vi "Global_usbComm.vi"() -> ()   [LabVIEW 2018]
panel:
  in  "Inspection Point":string
  in  "Specsheet Scan":string
  in  "PO Line Number":string
  in  "PO Number":string
  in  "Inspector":string="id:0"
  in  "Station":string
  in  "Serial Port":refnum<visa-resource-name>
  in  "Vendor Number":string
  in  "Vendor Name":string
  out "PIC_ARRAY":picture[](array[picture])=[bytes[1209480], bytes[921630], bytes[921630], bytes[346830], bytes[720330]]
  out "usbType":string
  out "Version":string[][](array[string])=[["Date", "Version", "Status", "Mod By"], ["20190701", "0", "Sic parvis magna", "id:0"], ["20191212", "1", "Successful test on 5 various consoles", "id:0"], ["20200125", "2", "Test for release", "id:0"], ["20200211", "3", "Fixed several bugs and rease for testing", "id:0"], ["20200213", "4", "Set foundation to handle Freemotion", "id:0"], ["20200214", "5", "Fixed small bugs", "id:0"], ["20200228", "6", "Changed reports so that all data will be visible with  SQL server", "id:0"], ["", "", "", ""]]
  in  "RS485_GearValues":dbl[][](array[numeric])=[[194.0, 245.0, 310.0, 375.0, 439.0, 504.0, 569.0, 634.0, 698.0, 763.0, 828.0, 892.0, 957.0, 1022.0, 1087.0, 1151.0, 1216.0, 1281.0, 1345.0, 1410.0, 1475.0, 1539.0, 0.0, 0.0, 0.0, 0.0], [194.0, 245.0, 310.0, 362.0, 427.0, 478.0, 543.0, 595.0, 659.0, 711.0, 776.0, 841.0, 892.0, 957.0, 1009.0, 1074.0, 1125.0, 1190.0, 1242.0, 1307.0, 1371.0, 1423.0, 1488.0, 1539.0, 0.0, 0.0], [194.0, 0.0, 0.0, 0.0, 0.0, 0.0, 0.0, 0.0, 0.0, 0.0, 0.0, 0.0, 0.0, 0.0, 0.0, 0.0, 0.0, 0.0, 0.0, 0.0, 0.0, 0.0, 0.0, 0.0, 0.0, 0.0]]
  out "resistanceType":string
  out "gradeType":string
  out "speedType":string
  out "tabletType":string
  in  "KeyCodes":string[][](array[string])=[["1", "2", "3", "4", "5", "6", "7", "8", "9", "10", "11", "12", "13", "14", "15", "", "", "", "", "", "", "", "", "", "", "", "", "", "", "", "", "", "", "", "", "", "", "", "", "", "", "", "", "", "", "", "", "", "", "", "", "", "", "", "", "", "", "", "", "", ""], ["1", "2", "3", "4", "5", "6", "7", "8", "9", "10", "11", "12", "13", "14", "15", "16", "17", "18", "19", "20", "21", "22", "23", "24", "", "", "", "", "", "", "", "", "", "", "", "", "", "", "", "", "", "", "", "", "", "", "", "", "", "", "", "", "", "", "", "", "", "", "", "", ""], ["-20", "-19", "-18", "-17", "-16", "-15", "-14", "-13", "-12", "-11", "-10", "-9", "-8", "-7", "-6", "-5", "-4", "-3", "-2", "-1", "0", "1", "2", "3", "4", "5", "6", "7", "8", "9", "10", "11", "12", "13", "14", "15", "16", "17", "18", "19", "20", "21", "22", "23", "24", "25", "26", "27", "28", "29", "30", "31", "32", "33", "34", "35", "36", "37", "38", "39", "40"], ["0", "1", "2", "3", "4", "5", "6", "7", "8", "9", "10", "11", "12", "13", "14", "15", "16", "17", "18", "19", "20", "21", "22", "23", "24", "25", "26", "27", "28", "29", "30", "", "", "", "", "", "", "", "", "", "", "", "", "", "", "", "", "", "", "", "", "", "", "", "", "", "", "", "", "", ""], ["1", "2", "3", "4", "5", "6", "7", "8", "9", "10", "11", "12", "13", "14", "15", "16", "17", "18", "19", "20", "21", "22", "23", "24", "25", "26", "27", "28", "29", "30", "31", "32", "", "", "", "", "", "", "", "", "", "", "", "", "", "", "", "", "", "", "", "", "", "", "", "", "", "", "", "", ""]]
  out "maxCurrent":string
  out "runCurrent":string
  out "fanType":string
  out "CALIBRATE- 9":string
  out "distanceType":string
  out "FINISH-25":string
  out "WAHOO-22":string
  out "CSAFE-21":string
  out "TV-20":string
  out "AUDIO-19":string
  out "FAN-18":string
  out "PULSE-17":string
  out "USB-16":string
  out "RESISTANCE-15":string
  out "INCLINE-14":string
  out "RPM-13":string
  out "PWM-12":string
  out "MAINTENANCE MODE-8, 9, 10, 11":string
  out "BLE_CONNECT-7":string
  out "POWER_UP-5, 6":string
  out "COSMETIC-3, 4":string
  out "BLE_SETUP-2":string
  out "FIXTURE_SETUP-1":string
  out "NEEDED-0":string
  out "PIP_Instruction":string[][](array[string])=[["", "FIXTURE_SETUP-1", "BLE_SETUP-2", "WARNING_LABEL-3", "COSMETIC-4", "POWER_UP-5", "DMK-6", "BLE_CONNECT-7", "SOFTWARE-8", "CALIBRATE-9", "DISPLAY-10", "KEY_PRESS-11", "PWM-12", "RPM-13", "INCLINE-14", "RESISTANCE-15", "USB-16", "PULSE-17", "FAN-18", "AUDIO-19", "TV-20", "CSAFE-21", "-22", "-23", "-24", "FINISH-25", "", "", "", ""], ["EQF1259 Console Fixture\nPC w/ Access to RNDftp\nMicroSD Card", "将EQW1001的一端连接到EQF1259（TRED1）。注意：确保您选择匹配控制台类型的正确端口。\n将接地线（绿色）连接到EQF 1259的E-GND。\nConnect one end of the EQW1001 to EQF1259 (TRED1). NOTE: MAKE SURE YOU SELECT THE CORRECT PORT THAT MATCH THE TYPE OF THE CONSOLE.   \nConnect the ground wire (Green) to E-GND on EQF 1259. \n", "打开测试平板电脑。\n点击iFit图标以启动应用程序。\n如果需要安装应用程序：\niFIT高级会员\n平板电脑/ iPad的Wi​​Fi连接\nBLE平板电脑应用设置：\n通过访问www.iFit.com加入iFit。\n购买/激活您的iFit高级会员。\n开启平板电脑的蓝牙功能。\n下载iFit蓝牙平板电脑应用程序。\n登录到您的iFit帐户并关闭弹出窗口。\n跳过设备配对，然后点击“了解”。\n注意：App的平板电脑/ iPad要求：\n•带有蓝牙4.0+的Android 5.0+\n•iPad 3及更高版本以及iOS 8+\n•屏幕宽度至少为600dp。 dp = px /（ppi / 160）\nTurn on test tablet.\nTap iFit icon to launch app.\nIf App Setup Needed:\nPremium iFIT Membership\nWiFi Connection For Tablet/iPad\nBLE Tablet App Setup:\nJoin iFit by visiting www.iFit.com.\nPurchase/Activate your iFit Premium Membership.\nTurn tablet Bluetooth ON.\nDownload the iFit Bluetooth Tablet App.\nSign into your iFit account and close popup windows.\nSkip the device pairing and tap “Got It”.\nNOTE: Tablet/iPad Requirements for App:\n• Android 5.0+ with Bluetooth 4.0+\n• iPad 3 and above with iOS 8+\n• A minimum of 600dp screen width.  dp = px / ( ppi / 160 )\n", "验证是否在控制台或脉冲条上打印了常规警告。 \nVerify that the General Warning is printed on the console or pulse bar.", "确认防静电袋是耗散的，并按照图纸打印。\n确保将设备包装在防静电袋中。\n目视检查控制台是否存在外观缺陷，物理损坏和难以辨认的打印。\n验证控制台匹配图片\nVerify that the ESD bag is dissipative and it is printed on as per the drawing.\nEnsure the unit is packaged in an antistatic bag. \nVisually inspect the console for cosmetic defects, physical damage, and illegible printing.  \nVerify console matches picture\n", "如果需要连接;脉冲条/手柄，扬声器，风扇，电视等。\n将8针MTA连接到控制台。\n单击确定。\nConnect if needed; pulse bar/grips, speakers, fans, TV, etc.\nConnect the 8-pin MTA to console.\nClick OK.", "将安全钥匙插入控制台。 \nInsert safety key into console.", "如果控制台显示Hello或ifit.com/activate，请按住iFit（SYNC）按钮10秒钟。\n在平板电脑上，触摸屏幕左上方的用户个人资料图标。\n在下拉列表中，触摸蓝牙。\n按下控制台上的iFIT同步按钮，并在显示屏中间验证4个字符的十六进制代码（示例：“ DF69”）。\n在弹出窗口中，验证与4个字符的十六进制代码匹配的控制台的信号强度为0.5m为（&gt; 50％）。\n连接到与4个字符的十六进制代码匹配的控制台。\n在控制台/装置上按开始。\nIf console displays  Hello or ifit.com/activate, press and hold the iFit (SYNC) button for 10 seconds.\nOn the tablet, touch user profile icon at the upper left  of the screen.\nIn drop down list, touch Bluetooth.\nPress the iFIT sync button on the console and verify a 4 character hex code in the middle of the display (Example: “DF69”). \nIn the pop up window, verify signal strength of the console that matches the 4 character hex code is at 0.5m is (&gt;50%).\nConnect to the console that matches the 4 character hex code.\nPress Start on console/fixture.", "如果控制台显示“欢迎”，请触摸iFit徽标。\n触摸跳过。\n触摸继续而不登录。\n触摸跳过。\n触摸屏幕左上方的用户个人资料图标。\n在下拉列表中，触摸设置。\n依次触摸设备信息和应用信息。这将显示App版本和Brainboard版本。\n验证并记录。\n返回设定画面。\n请注意，在平板电脑上进行的每个选择都由扬声器发出声音响应。\nIf console displays  WELCOME touch the iFit logo.\nTouch SKIP.\nTouch Continue without signing in.\nTouch SKIP.\nTouch user profile icon at the upper left  of the screen.\nIn drop down list, touch settings.\nTouch Equipment Info and then App Info. This will display App version and Brainboard version.\nVerify and Record.\nReturn to settings screen.\nNote that each selection made on the tablet was denoted with an audible response from the speakers.", "触摸维护。\n选择校准倾斜。\n在EQF1259上按Calibrate。\n在平板电脑上按开始以开始倾斜校准。确认显示屏上的倾斜值短暂增加，暂停，然后减小到零。\n校准完成后，返回设置屏幕。\n请注意，在平板电脑上进行的每个选择都由扬声器发出声音响应。\nTouch Maintenance.\nSelect Calibrate Incline.\nPress Calibrate on EQF1259.\nPress Begin on tablet to start incline calibration.  Verify the incline value on the display increases briefly, pauses, then decrease to zero.\nWhen calibration is complete, exit back to settings screen.\nNote that each selection made on the tablet was denoted with an audible response from the speakers.", "验证平板电脑显示屏是否亮起且没有缺陷 \nVerify tablet display is lit and without flaws.", "请注意，在平板电脑上进行的每个选择都带有扬声器发出的声音响应。\n返回主画面。\nNote that each selection made on the tablet was denoted with an audible response from the speakers.\nReturn to the main screen.", "在控制台上开始手动锻炼。\n在控制台上，按随机快速按钮。\n验证控制台和EQF1259上的速度是否匹配。\nStart manual workout on the console.\nOn the console, press random Quick speed buttons.\nVerify that the Speed on the console and EQF1259 match.", "在控制台上开始手动锻炼\n在EQF1259上按START（开始）。\n验证控制台上的Cadence（RPM）和EQF1259匹配。\nStart manual workout on the console\nOn the EQF1259, Press START.\nVerify that the Cadence(RPM) on the console and the EQF1259 match.", "在控制台上，按随机快速倾斜按钮。\n验证控制台上的倾斜和EQF1259匹配。\nOn the console, press random Quick incline buttons.\nVerify that the Incline on the console and EQF1259 match.", "在控制台上，按下RESISTANCE +按钮，确认EQF1259的电阻值增加。\n在控制台上，按RESISTANCE - 按钮。 验证EQF1259的电阻值是否下降。\nOn the console, press the RESISTANCE + button. Verify the resistance level on the EQF1259 increases.  \nOn the console, press the RESISTANCE - button. Verify the resistance level on the EQF1259 decreases.", "插入USB测试仪（注意红色加电压〜0V）。\n插入USB闪存驱动器（在USB测试仪上，插入闪存驱动器时，红色加电压约为3V，蓝色负电压将保持约为0V）。\n在USB测试仪上，绿色输出电压约为5Vdc。\n在USB测试仪上，蓝色输出电流约为30mA。\nPlug in USB tester (note the red plus voltage ~0V).\nPlug in the USB flash drive  (on the USB tester, red plus voltage ~3V when the flash drive is plugged in, blue negative voltage will stay ~0V).\nOn the USB tester, Green output voltage is ~5Vdc.\nOn the USB tester, Blue output current is ~30mA.", "握住脉冲棒/手柄\n在控制台上，确认显示了脉冲读数。\nHold the pulse bars/grips\nOn the console, verify a pulse reading is displayed.", "在控制台上，按大风扇按钮，风扇应在低速运行。\n在控制台上，再次按“大风扇”按钮，直到其高电平为止。\n在控制台上，按小风扇按钮，直到风扇关闭。\nOn the console, press the Large fan button and the fan should run on low.\nOn the console, press the Large fan button again until is on high.\nOn the console, press the Small fan button until the fan turns off.", "将EQW1007连接到音频源，并将EQW1007的另一端连接到控制台。\n在音频设备上，播放音频并验证其是否可以从两个控制台扬声器中播放。\n在控制台上，如果具有音量按钮，请调整到最小和最大级别并确认更改。\nConnect the EQW1007 to an audio source and connect the other end of the EQW1007 to the console.\nOn the audio device, play audio and verify that it plays out of both console speakers.\nOn the console, if it has volume buttons, adjust to minimum and maximum level and verify a change.", "将HDMI电缆连接到电视机。\n将HDMI电缆连接到控制台，控制台屏幕和声音将在电视上镜像。\nConnect the HDMI cable to the TV.\nConnect the HDMI cable to the console and the console screen and sound will be mirrored on the TV.", "将RJ45以太网电缆的一端连接到MYE CardioCare，另一端连接到控制台的背面\nMYE CardioCare模块上的电源和设备指示灯将亮起\nConnect one end of RJ45 ethernet cable to the MYE CardioCare and other end to back of console\nThe power and equipment indicators will light up on the MYE CardioCare module", "", " ", "", "触摸屏幕右下角的用户个人资料图标，清除缓存。\n触摸设置。\n触摸维护。\n轻触[清除应用程式快取]，然后选取[是]，就会出现[欢迎使用]。\n等待10秒钟，然后在EQF1259上关闭控制台电源。\n断开控制台上的所有电线和电缆。\nClear cache by touch the user profile icon on lower right of the screen.\nTouch Settings.\nTouch Maintainance.\nTouch Clear App Cache and select YES and WELCOME will appear on display.\nWait 10 seconds and then on the EQF1259, turn off the Console power.\nDisconnect all wires and cables from the console.", "", "", "", ""], ["EQW1141; 2-pin harness", "将EQW1025的一端连接到EQF1259（TRED2）。注意：确保您选择匹配控制台类型的正确端口。\n将接地线（绿色）连接到EQF 1259的E-GND。\nConnect one end of the EQW1025 to EQF1259 (TRED2). NOTE: MAKE SURE YOU SELECT THE CORRECT PORT THAT MATCH THE TYPE OF THE CONSOLE.   \nConnect the ground wire (Green) to E-GND on EQF 1259. ", "具有Ant +功能的Android手机或平板电脑，或带有Ant +软件狗和适配器的平板电脑。\n需要的应用程序：\nAnt +插件采样器\nANT +插件服务\nANT USB服务\nANT无线电服务\nAndroid phone or Tablet that is Ant+ capable or tablet with Ant+ dongle and adapter.\nApps Needed:\nAnt+ Plugins Sampler\nANT+ Plugins Services\nANT USB Service\nANT Radio Service\n", " ", "确认防静电袋是耗散的，并按照图纸打印。\n确保将设备包装在防静电袋中。\n目视检查控制台是否存在外观缺陷，物理损坏和难以辨认的打印。\n验证控制台匹配图片\n如果平板电脑有倾斜，请确认倾斜平稳移动，保持位置，并在整个范围内旋转。\nVerify that the ESD bag is dissipative and it is printed on as per the drawing.\nEnsure the unit is packaged in an antistatic bag. \nVisually inspect the console for cosmetic defects, physical damage, and illegible printing.  \nVerify console matches picture\nIf tablet has tilt, verify tilt  is smooth moving, holds position, and rotates through full range.", "如果需要连接;脉冲条/手柄，扬声器，风扇，电视等。\n将12针MTA连接到控制台。\n单击确定。\nConnect if needed; pulse bar/grips, speakers, fans, TV, etc.\nConnect the 12-pin MTA to console.\nClick OK.", " ", "按住暂停按钮5秒钟以获得Ant + ID。\n运行Ant + Sampler应用程序。\n从设备类型列表屏幕中选择“健身设备控制显示”。\n找到后，从步骤2中选择ID。\n如果询问，请选择不保存。\n您应该看到一个新的屏幕，其中包含跑步机数据。\n在控制台上按START。\nHold down pause button for 5 seconds to get Ant+ ID.\nRun Ant+ Sampler app.\nSelect ‘Fitness Equipment Controls Display’ from equipment type list screen.\nSelect the ID from step 2 when found.\nSelect Don’t Save if asked.\nYou should see a new screen with Treadmill data.\nPress START on the console.", "触摸屏幕下部中央的齿轮图标。\n触摸维护。这将显示App版本和Brainboard版本。\n验证并记录。\nTouch gear icon at the lower center  of the screen.\nTouch Maintainance. This will display App version and Brainboard version.\nVerify and Record.", "选择校准倾斜。\n在EQF1259上按Calibrate。\n在平板电脑上按开始以开始倾斜校准。确认显示屏上的倾斜值短暂增加，暂停，然后减小到零。\n校准完成后，返回设置屏幕。\nSelect Calibrate Incline.\nPress Calibrate on EQF1259.\nPress Begin on tablet to start incline calibration.  Verify the incline value on the display increases briefly, pauses, then decrease to zero.\nWhen calibration is complete, return to the settings screen.", " ", "选择键码。\n按下控制台上的所有按钮，每个按钮将显示一个唯一的代码。\n按平板电脑上的后退箭头以返回主屏幕。\nSelect Keycodes.\nPress all the buttons on the console and each will display a unique code.\nPress the back arrow on the tablet to return to main screen.", "", "在控制台上开始手动锻炼\n在EQF1259上，按START。\n验证控制台上的Cadence（RPM）和EQF1259是否匹配。\n验证控制台上的速度和EQF1259是否匹配。\nStart manual workout on the console\nOn the EQF1259, Press START.\nVerify that the Cadence(RPM) on the console and the EQF1259 match.\nVerify that the Speed on the console and the EQF1259 match.", " ", " ", "插入USB测试仪（注意红色加电压〜0V）。\n插入移动设备，它将指示正在充电（在USB测试仪上，插入闪存驱动器时，红色加电压约为3V，蓝色负电压将保持约为0V）。\n在USB测试仪上，绿色输出电压约为5Vdc。\n在USB测试仪上，蓝色输出电流约为2500mA。\nPlug in USB tester (note the red plus voltage ~0V).\nPlug in a mobile device and it will indicate charging  (on the USB tester, red plus voltage ~3V when the flash drive is plugged in, blue negative voltage will stay ~0V).\nOn the USB tester, Green output voltage is ~5Vdc.\nOn the USB tester, Blue output current is ~2500mA.", "在控制台上，按下拇指脉冲按钮上的拇指，并确认显示了脉冲读数。\nOn the console, press thumb onto the thumb pulse button and verify a pulse reading is displayed.", "将3针风扇连接到控制台。\n在控制台上，按“大风扇”按钮以打开风扇。风扇应在低位运行。\n再按一次“大风扇”按钮，直到它拉高。\n按下小风扇按钮，直到关闭风扇。\nConnect the 3-pin fans to the console.\nOn the console, press the Large Fan button to turn fan on. Fan should run on low.\nPress the Large Fan button again until is on high.\nPress the Small Fan button until it turns the fan off.", "在控制台上，连接耳机并将音量调到最小和最大，然后确认更改。\nOn the console, connect headphones and adjust volume to minimum and maximum and verify a change.", "将视频源连接到电视\n将EQWxxxx线束连接到电视机，另一端连接到控制台的背面\n将EQWxxxx线束连接到电视机，另一端连接到控制台的背面\n使用控制台控制开启电视机并在电视机上播放视频源\n音频将通过控制台扬声器播放\n在调音台上调节电视音频音量，该功能将显示在电视上，调音台音频将反映变化\nConnect video source to TV\nConnect EQWxxxx to the TV and other end to back of console\nConnect  EQWxxxx harness to the TV and other end to back of console\nTurn on TV with console controls and play video source on TV\nAudio will play through the console speakers\nAdjust TV audio volume on console and the function will display on the TV and the console audio will reflect change", " ", " ", " ", "", " ", "", "", "", ""], ["EQW1011; 3-pin harness", "将EQW1056的一端连接到EQF1259（TRED3）。注意：确保您选择匹配控制台类型的正确端口。\n将接地线（绿色）连接到EQF 1259的E-GND。\n按一次显示。\nConnect one end of the EQW1056 to EQF1259 (TRED3). NOTE: MAKE SURE YOU SELECT THE CORRECT PORT THAT MATCH THE TYPE OF THE CONSOLE.   \nConnect the ground wire (Green) to E-GND on EQF 1259. ", " ", " ", " ", "如果需要连接;脉冲条/手柄，扬声器，风扇，电视等。\n将4针MTA连接到控制台。\n单击确定。\nConnect if needed; pulse bar/grips, speakers, fans, TV, etc.\nConnect the 4-pin MTA to console.\nClick OK.", " ", " ", "在屏幕的外部边缘周围绘制一个矩形。\n触摸维护。这将显示App版本和Brainboard版本。\n验证并记录。\nDraw a rectangle around the outer edge of the screen.\nTouch Maintainance. This will display App version and Brainboard version.\nVerify and Record.", "", " ", "", "", "", "", "", "", "在胸带上，用拇指轻轻擦拭传感器\n在控制台上，将显示心律\nOn the chest strap, gently rub the sensors with your thumbs\nOn the console, a heart rate will display", " ", "在音频设备上，进入蓝牙设置屏幕。\n在控制台上，按住BLE按钮3秒钟。\n在音频设备上，与ifit Audio配对并播放音频。\n在控制台上，调节音量，音频电平将根据调节而改变。\n在音频设备上，进入蓝牙设置屏幕，然后断开连接并取消配对。\nOn the audio device, enter the bluetooth setup screen.\nOn the console, press and hold BLE button for 3 sec.\nOn audio device, Pair with ifit Audio and play audio.\nOn the console, adjust the volume and the audio level will change with respect to adjustment.\nOn audio device, enter the bluetooth setup screen and disconnect and unpair ifit Audio.", "将音频源连接到EQF1293并按播放\n将EQWxxxx公头直流电连接到公头直流电源适配器电缆，连接到EQF1293和控制台的其他端到端\n将RJ45以太网电缆的一端连接到EQF1293和控制台的另一端到后端\n将耳机连接到控制台并放在耳朵上\n按下控制台上的所有电视控制按钮，EQF1293上将显示响应\n音频将通过耳机播放\n在控制台上调整电视音频音量，该功能将显示在MYE电视上，耳机音频将反映变化 \nConnect EQWxxxx male dc to male dc power adapter cable to EQF1293 and other end to back of console\nConnect one end of RJ45 ethernet cable to the EQF1293 and other end to back of console\nPress all the TV control buttons on the console and a response will appear on the EQF1293", " ", " ", " ", "", "在EQF1259上，关闭控制台电源。\n断开控制台上的所有电线和电缆。\nOn the EQF1259, turn off the Console power.\nDisconnect all wires and cables from the console.", "", "", "", ""], ["EQW1059; 4-pin harness", "将EQW1053的一端连接到EQF1259（CLUB）。注意：确保您选择匹配控制台类型的正确端口。\n将接地线（绿色）连接到EQF 1259的E-GND。\nConnect one end of the EQW1053 to EQF1259 (CLUB). NOTE: MAKE SURE YOU SELECT THE CORRECT PORT THAT MATCH THE TYPE OF THE CONSOLE.   \nConnect the ground wire (Green) to E-GND on EQF 1259. ", " ", " ", " ", "如果需要连接;脉冲条/手柄，扬声器，风扇，电视等。\n将14针MTA连接到控制台。\n单击确定。\nConnect if needed; pulse bar/grips, speakers, fans, TV, etc.\nConnect the 14-pin MTA to console.\nClick OK.", " ", " ", "在卸下并重新插入安全钥匙的同时，按住“停止”按钮。\n验证并记录软件版本。\n通过“停止”按钮前进屏幕。\nPress and hold the Stop button while removing and re inserting the safety key.\nVerify and record software version.\nAdvance screen with button STOP.", "前进屏幕以进行校准。\n按校准按钮EQF1259\n按向上倾斜箭头以校准倾斜度。确认显示屏上的倾斜值短暂增加，暂停，然后减小到零。\nAdvance screen to incline calibrate.\nPress the Calibrate buttton the EQF1259\nPress Incline up arrow to calibrate incline. Verify the incline value on the display increases briefly, pauses, then decrease to zero.", "前进屏幕以显示测试。\n按向上倾斜箭头以空白并填充显示\n确认没有LCD段应暗淡，缺失，重影，闪烁或熄灭。\nAdvance screen to display test.\nPress Incline up arrow to blank and fill display\nVerify that there are no LCD segments should be dim, missing, ghosting, aglow, or out.", "进入屏幕进行按键测试。\n按下控制台上的所有按钮，每个按钮将显示一个唯一的代码。\n拉安全键返回到待机屏幕。\nAdvance screen to key test.\nPress all the buttons on the console and each will display a unique code.\nPull safety key to return to the idle screen.  ", "", "", "", "", "", "在灯具上，按开始按钮。\n在控制台上，点击“ IFIT同步”按钮。\n在控制台上，确认已显示生成的夹具脉冲。\nOn the fixture, press Start button.\nOn the console, tap the IFIT sync button.\nOn the console, verify that the generated fixture pulse is displayed.", " ", "将音频源连接到EQF1293并按播放\n将EQWxxxx公直流至公直流电源适配器电缆连接至EQF1293，另一端连接至控制台背面\n将RJ45以太网电缆的一端连接到EQF1293，另一端连接到控制台背面\n在控制台上，连接耳机并将音量调到最小和最大，然后确认更改。\nConnect audio source to EQF1293 and press play\nConnect EQWxxxx male dc to male dc power adapter cable to EQF1293 and other end to back of console\nConnect one end of RJ45 ethernet cable to the EQF1293 and other end to back of console\nOn the console, connect headphones and adjust volume to minimum and maximum and verify a change.", " ", " ", " ", " ", "", "按下并按住Ifit按钮（同步）并且速度增加和减少3秒钟以锁定控制台\n验证是否显示“”Hello“”或“”ifit.com/activate“”\n在EQF1259上，关闭控制台电源。\n断开控制台上的所有电线和电缆。\nLock console by press and holding the Ifit button (SYNC) and the Speed increase and decrease for 3 seconds\nVerify that Hello or ifit.com/activate is displayed\nOn the EQF1259, turn off the Console power.\nDisconnect all wires and cables from the console.", "", "", "", ""], ["EQW1067; 5-pin harness", "将EQW1001的一端连接到EQF1259（BOSTON1）。注意：确保您选择匹配控制台类型的正确端口。\n将接地线（绿色）连接到EQF 1259的E-GND。\nConnect one end of the EQW1001 to EQF1259 (BOSTON1). NOTE: MAKE SURE YOU SELECT THE CORRECT PORT THAT MATCH THE TYPE OF THE CONSOLE.   \nConnect the ground wire (Green) to E-GND on EQF 1259.", " ", " ", " ", " ", " ", " ", "插入安全键的同时按STOP按钮。\n按STOP次以查看软件。\n按SPEED UP按钮验证并记录屏幕上显示的V80.262或更高版本的软件。\n按SPEED UP按钮验证并记录软件部件号。\n按SPEED UP按钮以验证屏幕上显示的序列号。它应该与序列号标签上的序列号相同。\n按SPEED UP按钮验证并记录屏幕上显示的OLYMPUS板软件版本OLY 73。\n按SPEED UP按钮验证并记录屏幕W 1.15.1上显示的Wahoo开发板软件版本。\n按SPEED UP按钮验证并记录屏幕上显示的Bootloader软件版本3.1.4.5。\n按SPEED UP按钮验证并记录Wahoo ID号。\n按SPEED UP按钮验证并记录屏幕上显示的USB软件版本USB22。\n按STOP六次，然后按INCLINE UP以显示WAHOO。 （如果已经显示WAHOO，请按INCIN UP两次。这将启动收音机。）\n在平板电脑上打开ANT + Sampler应用程序。\n从设备类型列表屏幕中选择“健身设备控制显示”。\n从此控制台中选择ID。\n如果询问，请选择“不保存”。\n验证ID与该控制台中的ID匹配。\n通过“停止”按钮前进屏幕。\nPress the STOP button while inserting the SAFETY Key.\nPress STOP  times to view software.\nPress SPEED UP button toverify and record the software version V80.262 or greater showing on the screen.\nPress SPEED UP button toverify and record the software part number.\nPress SPEED UP button to verify the Serial Number showing on the screen. It should be the same as the serial number on the serial number sticker. \nPress SPEED UP button to verify and record the OLYMPUS board software version showing on the screen, OLY 73. \nPress SPEED UP button to verify and record the Wahoo board software version showing on the screen, W 1.15.1. \nPress SPEED UP button to verify and record the Bootloader software version showing on the screen, 3.1.4.5.\nPress SPEED UP button to verify and record the Wahoo ID number.\nPress SPEED UP button to verify and record the USB software version showing on the screen, USB22.\nPress STOP six times then press the INCLINE UP to display WAHOO. (If WAHOO is already displayed, press the INCLINE UP two times. This will initiate the radio.)\nOpen ANT+ Sampler app on the tablet.\nSelect 'Fitness Equipment Control Display' from equipment type list screen.\nSelect the ID from this console.\nSelect 'Don't Save' if asked.\nVerify that the ID matches the one from this console.\nAdvance screen with button STOP.", "", "前进屏幕，直到屏幕上显示OTF SYNC。\nOTF SYNC指示灯将打开，然后所有其他指示灯将打开和关闭。使用SPEED UP可以加快此过程。\n确认没有LCD段应变暗或变暗。\nAdvance screen till  OTF SYNC showing on the screen.\nOTF SYNC LED will turn on, and then all the other LED will turn on and off. Use SPEED UP to make this process quicker.\nVerify that there are no LCD segments should be dim or out.", "", "在控制台上，如果未运行，请按START\n在控制台上，按下一个“快速速度”按钮，然后等待结果直到指示灯保持点亮。\n在控制台上，按递减速度按钮，直到显示出来。\n在控制台上，按增量速度按钮，直到显示出来。\n在控制台上，按最低的“快速速度”按钮。\nOn the console, press START if not running\nOn the console, press next Quick speed button and wait for results till indicator remains lit.\nOn the console, press decrement speed button till indicated.\nOn the console, press increment speed button till indicated.\nOn the console, press the lowest Quick speed button.", "在固定装置上，如果未运行，请按开始\n验证控制台上的Cadence（RPM）和EQF1259是否匹配。\nOn the fixture, press START if not running\nVerify that the Cadence(RPM) on the console and the EQF1259 match.", "在控制台上，按下一个“快速倾斜”按钮，然后等待结果直到指示灯保持点亮。\n在控制台上，按减量倾斜按钮，直到显示出来。\n在控制台上，按增量倾斜按钮，直到显示出来。\n在控制台上，按最低的“快速倾斜”按钮。\nOn the console, press next Quick incline button and wait for results till indicator remains lit.\nOn the console, press decrement incline button till indicated.\nOn the console, press increment incline button till indicated.\nOn the console, press the lowest Quick incline button.", "在控制台上，按下下一个“快速电阻”按钮，然后等待结果直到指示灯保持点亮。\n在控制台上，按减阻按钮直到显示出来。\n在控制台上，按增加电阻按钮直到显示出来。\n在控制台上，按最低的“快速抵抗”按钮。\nOn the console, press next Quick resistance button and wait for results till indicator remains lit.\nOn the console, press decrement resistance button till indicated.\nOn the console, press increment resistance button till indicated.\nOn the console, press the lowest Quick resistance button.", "", "在灯具上，按开始按钮。\n在控制台上，确认已显示生成的夹具脉冲。\nOn the fixture, press Start button.\nOn the console, verify that the generated fixture pulse is displayed.", " ", " ", " ", " ", " ", " ", "", "按下并保持“Ifit”按钮（SYNC）和电阻（GEAR）增加和减少3秒钟以锁定控制台\n验证是否显示“你好”或“ifit.com/activate”\n在EQF1259上，关闭控制台电源。\n从控制台上取下电池\n断开控制台上的所有电线和电缆。 \nLock console by press and holding the Ifit button (SYNC) and the Resistance (GEAR) increase and decrease for 3 seconds\nVerify that Hello or ifit.com/activate is displayed\nOn the EQF1259, turn off the Console power.\nRemove batteries from console\nDisconnect all wires and cables from the console.", "", "", "", ""], ["EQW1001; 8-pin harness", "将EQW1025的一端连接到EQF1259（BOSTON2）。注意：确保您选择匹配控制台类型的正确端口。\n将接地线（绿色）连接到EQF 1259的E-GND。\nConnect one end of the EQW1025 to EQF1259 (BOSTON2). NOTE: MAKE SURE YOU SELECT THE CORRECT PORT THAT MATCH THE TYPE OF THE CONSOLE.   \nConnect the ground wire (Green) to E-GND on EQF 1259.", " ", " ", " ", "如果需要连接;脉冲条/手柄，扬声器，风扇，电视等。\n将2针MTA连接到控制台。\n将电池插入控制台，然后单击“确定”。\nConnect if needed; pulse bar/grips, speakers, fans, TV, etc.\nConnect the 2-pin MTA to console.\nInsert batteries into console and Click OK.", " ", " ", "在移除并重新插入安全钥匙的同时，按住Stop and Speed +按钮。\n验证并记录软件版本。\n通过“停止”按钮前进屏幕。\nPress and hold the Stop and Speed + button while removing and re inserting the safety key.\nVerify and record software version.\nAdvance screen with button STOP.", "", "", "", " ", "在固定装置上，如果未运行，请按开始\n验证控制台上的Cadence（RPM）是否与屏幕匹配。\n验证控制台上的“速度”是否与屏幕匹配。\nOn the fixture, press START if not running\nVerify that the Cadence(RPM) on the console matches the screen.\nVerify that the Speed on the console matches the screen.", " ", " ", " ", " ", " ", " ", " ", " ", " ", " ", "", " ", "", "", "", ""], ["EQW1139; 10-pin harness", "连接EQW1067 EQF1259（BIKE）的一端。注意：确保您选择匹配控制台类型的正确端口。\nConnect one end of the EQW1067 EQF1259 (BIKE). NOTE: MAKE SURE YOU SELECT THE CORRECT PORT THAT MATCH THE TYPE OF THE CONSOLE.", " ", " ", " ", "如果需要连接;脉冲条/手柄，扬声器，风扇，电视等。\n将3针MTA连接到控制台。\n将电池插入控制台，然后单击“确定”。\nConnect if needed; pulse bar/grips, speakers, fans, TV, etc.\nConnect the 3-pin MTA to console.\nInsert batteries into console and Click OK.", " ", " ", "按设置或齿轮图标按钮。\n验证并记录。\n根据您的覆盖，使用按钮UP ICON或DISPLAY或NEXT DISPLAY或PLAY ICON（DISPLAY）或DOT ICON（DISPLAY）或BLOCK ICON（DISPLAY）前进屏幕。\nPress the SETTINGS or Gear icon button.\nVerify and Record.\nAdvance screen with button UP ICON or DISPLAY or NEXT DISPLAY or PLAY ICON(DISPLAY) or DOT ICON(DISPLAY) or BLOCK ICON(DISPLAY), based on your overlay.", "", "前进屏幕以显示测试。\n两次按FAN UP或DISPLAY或MANUAL或AUDIO UP或AUDIO DOWN按钮以清除并填充所有片段，具体取决于叠加层。\n确认没有LCD段应暗淡，缺失，重影，闪烁或熄灭。\nAdvance screen to display test.\nPress button FAN UP or DISPLAY or MANUAL or AUDIO UP or AUDIO DOWN two times to clear and fill all segments, based on your overlay.\nVerify that there are no LCD segments should be dim, missing, ghosting, aglow, or out.", "进入屏幕进行关键测试。\n按下控制台上的所有按钮，每个按钮将显示一个唯一的代码\n前进屏幕，直到返回控制台空闲屏幕。\nAdvance screen to key test.\nPress all the buttons on the console and each will display a unique code\nAdvance screen till you return to the console idle screen.", " ", "", " ", " ", " ", " ", " ", " ", " ", " ", " ", " ", "", " ", "", "", "", ""], ["EQW1139; 10-pin harness", "连接EQW1139 EQF1259（BIKE1）的一端。注意：确保您选择匹配控制台类型的正确端口。\nConnect one end of the EQW1139 EQF1259 (BIKE1). NOTE: MAKE SURE YOU SELECT THE CORRECT PORT THAT MATCH THE TYPE OF THE CONSOLE.", " ", " ", " ", "如果需要连接;脉冲条/手柄，扬声器，风扇，电视等。\n将5针MTA连接到控制台。\n将电池插入控制台，然后单击“确定”。\nConnect if needed; pulse bar/grips, speakers, fans, TV, etc.\nConnect the 5-pin MTA to console.\nInsert batteries into console and Click OK.", " ", " ", "按下ON_RESET或DISPLAY按钮。\n验证并记录。\n根据您的叠加，使用“失重”或“ CALORIE”或14个“ APPS”或“ TEMPO” APPS或1前进屏幕。\nPress the ON_RESET or DISPLAY  button.\nVerify and Record.\nAdvance screen with WEIGHT LOSS or CALORIE or 14 APPS or  TEMPO APPS or 1, based on your overlay.", " ", "高级屏幕显示测试。\n两次按下按钮““ FAN UP””或“ DISPLAY”或“ MANUAL”或“ AUDIO UP”或“ AUDIO DOWN”或“ GEAR PLUS ICON”或“ 6” 根据您的叠加层清除并填充所有细分。\n确认没有LCD分段应变暗，缺失，重影，闪烁或熄灭。\nAdvance screen to display test.\nPress button FAN UP or DISPLAY or MANUAL or AUDIO UP or AUDIO DOWN or GEAR PLUS ICON or 6 two times to clear and fill all segments, based on your overlay.\nVerify that there are no LCD segments should be dim, missing, ghosting, aglow, or out.", " ", " ", "", " ", " ", " ", " ", " ", " ", " ", " ", " ", " ", "", " ", "", "", "", ""], ["EQW1053; 14针线束 \nEQW1053; 14-pin harness", "将EQW1001的一端连接到EQF1259（BIKE2）。注意：确保您选择匹配控制台类型的正确端口。\n将VDC适配器的一端连接到EQF1259的CONSOLE插座。\nConnect one end of the EQW1001 to EQF1259 (BIKE2). NOTE: MAKE SURE YOU SELECT THE CORRECT PORT THAT MATCH THE TYPE OF THE CONSOLE.\nConnect one end of the VDC adapter to CONSOLE socket on the EQF1259.", " ", " ", " ", "必要时连接；脉冲条/手柄，扬声器，风扇，电视等\n将8针MTA连接到控制台。\n如果使用电池测试控制台，请在安装电池之前绝对确保控制台电源开关已关闭并且电池电压良好。用电池测试一半样品。请参阅警告。\n警告！请勿在控制台电源打开的情况下将电池安装到控制台中！这可能会导致电池充电和爆炸。\n警告！请勿安装总电压小于2伏的电池。这可能会导致电池充电和爆炸。\n电池测试：安装电池后，无论控制台开关处于什么位置，控制台电源LED都会亮起，表明控制台已通电。\n当打开控制台电源开关时，EQF1259检查控制台电压线，如果检测到2伏以上，则EQF1259假定控制台由电池供电，并且未打开控制台电压线的电源。单词“ Bat”将出现在显示屏的右上角，EQF1259将向控制台提供信号。\nVDC适配器测试：将VDC适配器连接到控制台\n单击确定。\nConnect if needed; pulse bar/grips, speakers, fans, TV, etc.\nConnect the 8-pin MTA to console.\nIf testing a console with batteries, be absolutely sure the console power switch is off before installing batteries and that the batteries have a good voltage.   Test half sample with batteries. See warnings. \nWarning!  DO NOT INSTALL BATTERIES INTO A CONSOLE WITH THE CONSOLE POWER SWITCH ON!  THIS MAY CAUSE BATTERIES TO CHARGE AND EXPLODE.\nWarning!  DO NOT INSTALL BATTERIES THAT HAVE A COMBINED VOLTAGE LESS THAN 2 VOLTS. THIS MAY CAUSE BATTERIES TO CHARGE AND EXPLODE.\nBattery test: Once batteries are installed, the Console Power LED will light regardless of the console switch position indicating the console had power. \nWhen turning on the console power switch, the EQF1259 checks the console voltage line and if more than 2 volts is detected, the EQF1259 assumes the console is powered by batteries and does not turn on power to the console voltage wires.  The word “Bat” will appear in the top right corner of the display and the EQF1259 will provide signals to the console.\nVDC adapter test: Connect the VDC adapter to console\nClick OK.", " ", " ", "插入安全键的同时按STOP按钮。\n按STOP次以查看软件。\n按下SPEED UP按钮以验证并记录屏幕上显示的V80.262或更高版本的软件。\n按下SPEED UP按钮以验证并记录软件部件号。\n按SPEED UP按钮以验证屏幕上显示的序列号。它应该与序列号标签上的序列号相同。\n按SPEED UP按钮以验证并记录屏幕上显示的OLYMPUS板软件版本OLY 73。\n按SPEED UP按钮以验证并记录屏幕上显示的USB软件版本USB22。\n通过“停止”按钮前进屏幕。\nPress the STOP button while inserting the SAFETY Key.\nPress STOP  times to view software.\nPress SPEED UP button toverify and record the software version V80.262 or greater showing on the screen.\nPress SPEED UP button toverify and record the software part number.\nPress SPEED UP button to verify the Serial Number showing on the screen. It should be the same as the serial number on the serial number sticker. \nPress SPEED UP button to verify and record the OLYMPUS board software version showing on the screen, OLY 73. \nPress SPEED UP button to verify and record the USB software version showing on the screen, USB22.\nAdvance screen with button STOP.", "", "", "", " ", " ", " ", " ", " ", " ", " ", " ", " ", " ", " ", " ", "", " ", "", "", "", ""], ["EQW1189； WST 10针至8针MTA线束\nEQW1189; WST 10-pin to 8-pin mta harness", "将EQW1025的一端连接到EQF1259（椭圆）。注意：确保您选择匹配控制台类型的正确端口。\nConnect one end of the EQW1025 to EQF1259 (ELLIPTICAL). NOTE: MAKE SURE YOU SELECT THE CORRECT PORT THAT MATCH THE TYPE OF THE CONSOLE.", " ", " ", " ", "必要时连接；脉冲条/手柄，扬声器，风扇，电视等\n将10针MTA连接到控制台。\n如果使用电池测试控制台，请在安装电池之前绝对确保控制台电源开关已关闭并且电池电压良好。用电池测试一半样品。请参阅警告。\n警告！请勿在控制台电源打开的情况下将电池安装到控制台中！这可能会导致电池充电和爆炸。\n警告！请勿安装总电压小于2伏的电池。这可能会导致电池充电和爆炸。\n电池测试：安装电池后，无论控制台开关处于什么位置，控制台电源LED都会亮起，表明控制台已通电。\n当打开控制台电源开关时，EQF1259检查控制台电压线，如果检测到2伏以上，则EQF1259假定控制台由电池供电，并且未打开控制台电压线的电源。单词“ Bat”将出现在显示屏的右上角，EQF1259将向控制台提供信号。\n单击确定。\nConnect if needed; pulse bar/grips, speakers, fans, TV, etc.\nConnect the 10-pin MTA to console.\nIf testing a console with batteries, be absolutely sure the console power switch is off before installing batteries and that the batteries have a good voltage.   Test half sample with batteries. See warnings. \nWarning!  DO NOT INSTALL BATTERIES INTO A CONSOLE WITH THE CONSOLE POWER SWITCH ON!  THIS MAY CAUSE BATTERIES TO CHARGE AND EXPLODE.\nWarning!  DO NOT INSTALL BATTERIES THAT HAVE A COMBINED VOLTAGE LESS THAN 2 VOLTS. THIS MAY CAUSE BATTERIES TO CHARGE AND EXPLODE.\nBattery test: Once batteries are installed, the Console Power LED will light regardless of the console switch position indicating the console had power. \nWhen turning on the console power switch, the EQF1259 checks the console voltage line and if more than 2 volts is detected, the EQF1259 assumes the console is powered by batteries and does not turn on power to the console voltage wires.  The word “Bat” will appear in the top right corner of the display and the EQF1259 will provide signals to the console.\nClick OK.", " ", " ", "按下POWER GLYPH按钮。\n验证并记录。\nPress the POWER GLYPH button.\nVerify and Record.", "", "确认没有LCD段应变暗或变暗。\nVerify that there are no LCD segments should be dim or out.", "按下所有按钮，确认它们发出哔哔声。\nPress all buttons and verify that they beep.\n", " ", " ", " ", " ", " ", " ", " ", " ", " ", " ", " ", " ", "", " ", "", "", "", ""], ["安全钥匙 \nSafety Key", "将EQW1056的一端连接到EQF1259（RS-485）。注意：确保您选择匹配控制台类型的正确端口。\nConnect one end of the EQW1056 to EQF1259 (RS-485). NOTE: MAKE SURE YOU SELECT THE CORRECT PORT THAT MATCH THE TYPE OF THE CONSOLE.   ", " ", " ", " ", " ", " ", " ", " ", " ", " ", " ", " ", " ", " ", " ", " ", " ", " ", " ", " ", " ", " ", " ", "", " ", "", "", "", ""], ["iOS或Android平板电脑瓦特/最新的iFit应用程序 \niOS or Android Tablet w/ Latest iFit app ", "将EQW1053的一端连接到EQF1259（CLUB）。注意：确保您选择匹配控制台类型的正确端口。\nConnect one end of the EQW1053 to EQF1259 (CLUB). NOTE: MAKE SURE YOU SELECT THE CORRECT PORT THAT MATCH THE TYPE OF THE CONSOLE.", " ", " ", " ", " ", " ", " ", "插入安全键的同时按STOP按钮。 （仅29818）\n按停止按钮3次。\n按SPEED UP按钮以验证型号。\n按下SPEED UP按钮以验证屏幕上显示的软件版本V83.77或更高。\n按SPEED UP按钮以验证并记录软件部件号。\n按SPEED UP按钮以验证并记录屏幕上显示的USB软件版本USB22。\n按SPEED UP按钮以验证并记录屏幕上显示的BLE软件版本？。\n按SPEED UP按钮以验证屏幕上显示的序列号。它应该与序列号标签上的序列号相同。\n按SPEED UP按钮以验证并记录屏幕上显示的OLYMPUS板软件版本OLY 73。\nPress the STOP button while inserting the SAFETY Key. (29818 only)\nPress SPEED UP button to verify the model number.\nPress SPEED UP button to verify the software version V83.77 or greater showing on the screen.\nPress SPEED UP button to verify and record the software part number.\nPress SPEED UP button to verify and record the USB software version showing on the screen, USB22.\nPress SPEED UP button to verify and record the BLE software version showing on the screen, ?.\nPress SPEED UP button to verify the Serial Number showing on the screen. It should be the same as the serial number on the serial number sticker. \nPress SPEED UP button to verify and record the OLYMPUS board software version showing on the screen, OLY 73.\nAdvance screen with button STOP.", "", "前进屏幕以显示测试。\n按INCLINE˅按钮切换显示的开/关。\nAdvance screen to display test.\nPress INCLINE ˅ button to toggle display on/off.", "", " ", " ", " ", " ", " ", " ", " ", " ", " ", " ", " ", " ", "", " ", "", "", "", ""], ["EQWxxxx; MicroUSB电缆 \nEQWxxxx; MicroUSB Cable", "将EQW1011的一端连接到EQF1259（TACH1）。注意：确保您选择匹配控制台类型的正确端口。\nConnect one end of the EQW1011 to EQF1259 (TACH1). NOTE: MAKE SURE YOU SELECT THE CORRECT PORT THAT MATCH THE TYPE OF THE CONSOLE.\n", " ", " ", " ", " ", " ", " ", " ", " ", " ", " ", " ", " ", " ", " ", " ", " ", " ", " ", " ", " ", " ", " ", "", " ", "", "", "", ""], ["EQWxxxx; HDMI电缆带电视 \nEQWxxxx; HDMI Cable w/ TV", "将EQW1041的一端连接到EQF1259（TACH2）。注意：确保您选择匹配控制台类型的正确端口。\nConnect one end of the EQW1041 to EQF1259 (TACH2). NOTE: MAKE SURE YOU SELECT THE CORRECT PORT THAT MATCH THE TYPE OF THE CONSOLE.", " ", " ", " ", " ", " ", " ", " ", " ", " ", " ", " ", " ", " ", " ", " ", " ", " ", " ", " ", " ", " ", " ", "", " ", "", "", "", ""], ["极地脉冲带 \nPolar Pulse Strap", "将EQWxxxx公直流至公直流电源适配器电缆连接到EQF1259（CONSOLE）。注意：确保您选择匹配控制台类型的正确端口。\nConnect EQWxxxx male dc to male dc power adapter cable  to EQF1259 (CONSOLE). NOTE: MAKE SURE YOU SELECT THE CORRECT PORT THAT MATCH THE TYPE OF THE CONSOLE.", " ", " ", " ", "如果需要连接;脉冲条/手柄，扬声器，风扇，电视等。\n将EQWxxxx公头直流电源连接到公头直流电源适配器电缆连接到控制台背面。\n单击确定。\nConnect if needed; pulse bar/grips, speakers, fans, TV, etc.\nConnect EQWxxxx male dc to male dc power adapter cable to the back of the console.\nClick OK.", " ", " ", " ", " ", " ", " ", " ", " ", " ", " ", " ", " ", " ", " ", " ", " ", " ", " ", "", " ", "", "", "", ""], ["ANT +脉冲带 \nANT+ Pulse strap", "将EQW1084的一端连接到EQF1259（RS-485）。注意：确保您选择匹配控制台类型的正确端口。\nConnect one end of the EQW1084 to EQF1259 (RS-485). NOTE: MAKE SURE YOU SELECT THE CORRECT PORT THAT MATCH THE TYPE OF THE CONSOLE.", " ", " ", " ", "如有需要，请连接；脉冲条/手柄，扬声器，风扇，电视等。\n将6针DIN连接到控制台上的插座。\n将8针DIN连接到控制台上的插座。\n单击确定。\nConnect if needed; pulse bar/grips, speakers, fans, TV, etc.\nConnect the 6-pin DIN to the socket on the console.\nConnect the 8-pin DIN to the socket on the  console.\nClick OK.\n", " ", " ", " ", " ", " ", " ", " ", " ", " ", " ", " ", " ", " ", " ", " ", " ", " ", " ", "", " ", "", "", "", ""], ["iOS音频设备\nEQW1007; Auxillary Audio cable w/ iOS Audio Device", "将EQW1189的一端连接到EQF1259（BOSTON1）。注意：确保您选择匹配控制台类型的正确端口。\nConnect one end of the EQW1189 to EQF1259 (BOSTON1). NOTE: MAKE SURE YOU SELECT THE CORRECT PORT THAT MATCH THE TYPE OF THE CONSOLE.", " ", " ", " ", "如果需要连接;脉冲杆/把手，扬声器，风扇，电视等\n将RJ45连接器连接到控制台。\n单击确定。\nConnect if needed; pulse bar/grips, speakers, fans, TV, etc.\nConnect the RJ45 connector to console.\nClick OK.", " ", " ", " ", " ", " ", " ", " ", " ", " ", " ", " ", " ", " ", " ", " ", " ", " ", " ", "", " ", "", "", "", ""], ["EQW1007; 带有iOS音频设备的辅助音频电缆 \nMYE Audio Reciever w/ RJ45 Cable", "将EQW1139的一端连接到EQF1259（BIKE1）。注意：确保您选择匹配控制台类型的正确端口。\n将EQW1056的一端连接到EQF1259（RS-485）。注意：确保您选择匹配控制台类型的正确端口。 （对于加速度计速度）。\nConnect one end of the EQW1139 to EQF1259 (BIKE1). NOTE: MAKE SURE YOU SELECT THE CORRECT PORT THAT MATCH THE TYPE OF THE CONSOLE.\nConnect one end of the EQW1056 to EQF1259(RS-485). NOTE: MAKE SURE YOU SELECT THE CORRECT PORT THAT MATCH THE TYPE OF THE CONSOLE. (For Accelerometer Speed).", " ", " ", " ", "必要时连接；脉冲条/手柄，扬声器，风扇，电视等\n将10针MTA连接到控制台。\n将4针MTA连接到控制台。\n如果使用电池测试控制台，请在安装电池之前绝对确保控制台电源开关已关闭并且电池电压良好。用电池测试一半样品。请参阅警告。\n警告！请勿在控制台电源打开的情况下将电池安装到控制台中！这可能会导致电池充电和爆炸。\n警告！请勿安装总电压小于2伏的电池。这可能会导致电池充电和爆炸。\n电池测试：安装电池后，无论控制台开关处于什么位置，控制台电源LED都会亮起，表明控制台已通电。\n当打开控制台电源开关时，EQF1259检查控制台电压线，如果检测到2伏以上，则EQF1259假定控制台由电池供电，并且未打开控制台电压线的电源。单词“ Bat”将出现在显示屏的右上角，EQF1259将向控制台提供信号。\n单击确定。\nConnect if needed; pulse bar/grips, speakers, fans, TV, etc.\nConnect the 10-pin MTA to console.\nConnect the 4-pin MTA to the console.\nIf testing a console with batteries, be absolutely sure the console power switch is off before installing batteries and that the batteries have a good voltage.   Test half sample with batteries. See warnings. \nWarning!  DO NOT INSTALL BATTERIES INTO A CONSOLE WITH THE CONSOLE POWER SWITCH ON!  THIS MAY CAUSE BATTERIES TO CHARGE AND EXPLODE.\nWarning!  DO NOT INSTALL BATTERIES THAT HAVE A COMBINED VOLTAGE LESS THAN 2 VOLTS. THIS MAY CAUSE BATTERIES TO CHARGE AND EXPLODE.\nBattery test: Once batteries are installed, the Console Power LED will light regardless of the console switch position indicating the console had power. \nWhen turning on the console power switch, the EQF1259 checks the console voltage line and if more than 2 volts is detected, the EQF1259 assumes the console is powered by batteries and does not turn on power to the console voltage wires.  The word “Bat” will appear in the top right corner of the display and the EQF1259 will provide signals to the console.\nClick OK.", " ", " ", " ", " ", " ", " ", " ", " ", " ", " ", " ", " ", " ", " ", " ", " ", " ", " ", "", " ", "", "", "", ""], ["MYE音频接收器，带RJ45电缆 \nCardioCare WiFi Module w/ RJ45 Cable", "将EQW1025的一端连接到EQF1259（椭圆）。注意：确保您选择匹配控制台类型的正确端口。\n将EQW1056的一端连接到EQF1259（RS-485）。注意：确保您选择匹配控制台类型的正确端口。 （对于加速度计速度）。\nConnect one end of the EQW1025 to EQF1259 (ELLIPTICAL). NOTE: MAKE SURE YOU SELECT THE CORRECT PORT THAT MATCH THE TYPE OF THE CONSOLE.\nConnect one end of the EQW1056 to EQF1259(RS-485). NOTE: MAKE SURE YOU SELECT THE CORRECT PORT THAT MATCH THE TYPE OF THE CONSOLE. (For Accelerometer Speed).", " ", " ", " ", "如果需要，请连接；脉冲条/手柄，扬声器，风扇，电视等。\n将12针MTA连接到控制台。\n将4针MTA连接到控制台。\n单击确定。\nConnect if needed; pulse bar/grips, speakers, fans, TV, etc.\nConnect the 12-pin MTA to console.\nConnect the 4-pin MTA to the console.\nClick OK.", " ", " ", " ", " ", " ", " ", " ", " ", " ", " ", " ", " ", " ", " ", " ", " ", " ", " ", "", " ", "", "", "", ""], ["MYE电视\nRJ45电缆\nDC转直流适配器\n带同轴电缆的模拟视频源\nMYE TV\nRJ45 Cable\nDC to DC Adapter\nAnalog Video Source w/ Coax Cable", "\n将EQW1185的一端连接到EQF1259（BIKE1）。注意：确保您选择匹配控制台类型的正确端口。\nConnect one end of the EQW1185 to EQF1259 (BIKE1). NOTE: MAKE SURE YOU SELECT THE CORRECT PORT THAT MATCH THE TYPE OF THE CONSOLE.", " ", " ", " ", " ", " ", " ", " ", " ", " ", " ", " ", " ", " ", " ", " ", " ", " ", " ", " ", " ", " ", " ", "", " ", "", "", "", ""], ["将电源线连接到EQF1259。\n设置灯具配置：\n使用PC将.xml配置文件加载到microSD卡中，该文件在RNDftp中的控制台名称下找到（例如：…RNDFtp \\ EBNT02117 \\ Procedure）。\n将microSD卡面朝上插入microSD卡插槽中。\n打开灯具背面的RESET按钮。\n使用向上和向下按钮找到正确的配置文件。\n按ENTER选择配置文件（屏幕1）。\n当屏幕稳定时，请等待5秒钟，如下所示。\n设置夹具脉冲：\n按EQF1259 2x上的Display。\n在此灯具上按开始\n使用向上和向下按钮设置随机脉冲。\n在灯具上按开始。\n按一次显示。\nConnect the power cord to the EQF1259.\nSet Fixture Configurations:\nUsing PC, load .xml configuration file, which is found in the RNDftp under the console name (Example: …RNDFtp\\EBNT02117\\Procedure) to the microSD card.\nInsert the microSD card face up into the microSD card slot.\nTurn on the RESET button at the back of the fixture.\nUsing the UP and DOWN buttons locate the proper configuration file.\nPress ENTER to select the configuration file (Screen 1).\nWait for 5 seconds, when the screen is stable as below.\nSet Fixture Pulse:\nPress Display on the EQF1259 2x.\nPress Start on this fixture\nUsing the up and down buttons, set a random pulse.\nPress Start on the fixture.\nPress Display once.", " ", " ", " ", " ", " ", " ", " ", " ", " ", " ", " ", " ", " ", " ", " ", " ", " ", " ", " ", " ", " ", " ", " ", "", " ", "", "", "", ""], [" ", " ", " ", " ", " ", " ", " ", " ", " ", " ", " ", " ", " ", " ", " ", " ", " ", " ", " ", " ", " ", " ", " ", " ", "", " ", "", "", "", ""], [" ", " ", " ", " ", " ", " ", " ", " ", " ", " ", " ", " ", " ", " ", " ", " ", " ", " ", " ", " ", " ", " ", " ", " ", "", " ", "", "", "", ""], [" ", " ", " ", " ", " ", " ", " ", " ", " ", " ", " ", " ", " ", " ", " ", " ", " ", " ", " ", " ", " ", " ", " ", " ", "", " ", "", "", "", ""], [" ", " ", " ", " ", " ", " ", " ", " ", " ", " ", " ", " ", " ", " ", " ", " ", " ", " ", " ", " ", " ", " ", " ", " ", "", " ", "", "", "", ""], [" ", " ", " ", " ", " ", " ", " ", " ", " ", " ", " ", " ", " ", " ", " ", " ", " ", " ", " ", " ", " ", " ", " ", " ", "", " ", "", "", "", ""], [" ", " ", " ", " ", " ", " ", " ", " ", " ", " ", " ", " ", " ", " ", " ", " ", " ", " ", " ", " ", " ", " ", " ", " ", "", " ", "", "", "", ""], [" ", " ", " ", " ", " ", " ", " ", " ", " ", " ", " ", " ", " ", " ", " ", " ", " ", " ", " ", " ", " ", " ", " ", " ", "", " ", "", "", "", ""], [" ", " ", " ", " ", " ", " ", " ", " ", " ", " ", " ", " ", " ", " ", " ", " ", " ", " ", " ", " ", " ", " ", " ", " ", "", " ", "", "", "", ""], [" ", " ", " ", " ", " ", " ", " ", " ", " ", " ", " ", " ", " ", " ", " ", " ", " ", " ", " ", " ", " ", " ", " ", " ", "", " ", "", "", "", ""], [" ", " ", " ", " ", " ", " ", " ", " ", " ", " ", " ", " ", " ", " ", " ", " ", " ", " ", " ", " ", " ", " ", " ", " ", "", " ", "", "", "", ""], [" ", " ", " ", " ", " ", " ", " ", " ", " ", " ", " ", " ", " ", " ", " ", " ", " ", " ", " ", " ", " ", " ", " ", " ", "", " ", "", "", "", ""], [" ", " ", " ", " ", " ", " ", " ", " ", " ", " ", " ", " ", " ", " ", " ", " ", " ", " ", " ", " ", " ", " ", " ", " ", "", " ", "", "", "", ""], [" ", " ", " ", " ", " ", " ", " ", " ", " ", " ", " ", " ", " ", " ", " ", " ", " ", " ", " ", " ", " ", " ", " ", " ", "", " ", "", "", "", ""], [" ", " ", " ", " ", " ", " ", " ", " ", " ", " ", " ", " ", " ", " ", " ", " ", " ", " ", " ", " ", " ", " ", " ", " ", "", " ", "", "", "", ""], [" ", " ", " ", " ", " ", " ", " ", " ", " ", " ", " ", " ", " ", " ", " ", " ", " ", " ", " ", " ", " ", " ", " ", " ", "", " ", "", "", "", ""], [" ", " ", " ", " ", " ", " ", " ", " ", " ", " ", " ", " ", " ", " ", " ", " ", " ", " ", " ", " ", " ", " ", " ", " ", "", " ", "", "", "", ""], [" ", " ", " ", " ", " ", " ", " ", " ", " ", " ", " ", " ", " ", " ", " ", " ", " ", " ", " ", " ", " ", " ", " ", " ", "", " ", "", "", "", ""], [" ", " ", " ", " ", " ", " ", " ", " ", " ", " ", " ", " ", " ", " ", " ", " ", " ", " ", " ", " ", " ", " ", " ", " ", "", " ", "", "", "", ""], [" ", " ", " ", " ", " ", " ", " ", " ", " ", " ", " ", " ", " ", " ", " ", " ", " ", " ", " ", " ", " ", " ", " ", " ", "", " ", "", "", "", ""], [" ", " ", " ", " ", " ", " ", " ", " ", " ", " ", " ", " ", " ", " ", " ", " ", " ", " ", " ", " ", " ", " ", " ", " ", "", " ", "", "", "", ""], [" ", " ", " ", " ", " ", " ", " ", " ", " ", " ", " ", " ", " ", " ", " ", " ", " ", " ", " ", " ", " ", " ", " ", " ", "", " ", "", "", "", ""], [" ", " ", " ", " ", " ", " ", " ", " ", " ", " ", " ", " ", " ", " ", " ", " ", " ", " ", " ", " ", " ", " ", " ", " ", "", " ", "", "", "", ""], [" ", " ", " ", " ", " ", " ", " ", " ", " ", " ", " ", " ", " ", " ", " ", " ", " ", " ", " ", " ", " ", " ", " ", " ", "", " ", "", "", "", ""], [" ", " ", " ", " ", " ", " ", " ", " ", " ", " ", " ", " ", " ", " ", " ", " ", " ", " ", " ", " ", " ", " ", " ", " ", "", " ", "", "", "", ""], [" ", " ", " ", " ", " ", " ", " ", " ", " ", " ", " ", " ", " ", " ", " ", " ", " ", " ", " ", " ", " ", " ", " ", " ", "", " ", "", "", "", ""], [" ", " ", " ", " ", " ", " ", " ", " ", " ", " ", " ", " ", " ", " ", " ", " ", " ", " ", " ", " ", " ", " ", " ", " ", "", " ", "", "", "", ""], [" ", " ", " ", " ", " ", " ", " ", " ", " ", " ", " ", " ", " ", " ", " ", " ", " ", " ", " ", " ", " ", " ", " ", " ", "", " ", "", "", "", ""], [" ", " ", " ", " ", " ", " ", " ", " ", " ", " ", " ", " ", " ", " ", " ", " ", " ", " ", " ", " ", " ", " ", " ", " ", "", " ", "", "", "", ""], [" ", " ", " ", " ", " ", " ", " ", " ", " ", " ", " ", " ", " ", " ", " ", " ", " ", " ", " ", " ", " ", " ", " ", " ", "", " ", "", "", "", ""], [" ", " ", " ", " ", " ", " ", " ", " ", " ", " ", " ", " ", " ", " ", " ", " ", " ", " ", " ", " ", " ", " ", " ", " ", "", " ", "", "", "", ""], [" ", " ", " ", " ", " ", " ", " ", " ", " ", " ", " ", " ", " ", " ", " ", " ", " ", " ", " ", " ", " ", " ", " ", " ", "", " ", "", "", "", ""], [" ", " ", " ", " ", " ", " ", " ", " ", " ", " ", " ", " ", " ", " ", " ", " ", " ", " ", " ", " ", " ", " ", " ", " ", "", " ", "", "", "", ""], [" ", " ", " ", " ", " ", " ", " ", " ", " ", " ", " ", " ", " ", " ", " ", " ", " ", " ", " ", " ", " ", " ", " ", " ", "", " ", "", "", "", ""], [" ", " ", " ", " ", " ", " ", " ", " ", " ", " ", " ", " ", " ", " ", " ", " ", " ", " ", " ", " ", " ", " ", " ", " ", "", " ", "", "", "", ""], [" ", " ", " ", " ", " ", " ", " ", " ", " ", " ", " ", " ", " ", " ", " ", " ", " ", " ", " ", " ", " ", " ", " ", " ", "", " ", "", "", "", ""], [" ", " ", " ", " ", " ", " ", " ", " ", " ", " ", " ", " ", " ", " ", " ", " ", " ", " ", " ", " ", " ", " ", " ", " ", "", " ", "", "", "", ""], [" ", " ", " ", " ", " ", " ", " ", " ", " ", " ", " ", " ", " ", " ", " ", " ", " ", " ", " ", " ", " ", " ", " ", " ", "", " ", "", "", "", ""], [" ", " ", " ", " ", " ", " ", " ", " ", " ", " ", " ", " ", " ", " ", " ", " ", " ", " ", " ", " ", " ", " ", " ", " ", "", " ", "", "", "", ""], [" ", " ", " ", " ", " ", " ", " ", " ", " ", " ", " ", " ", " ", " ", " ", " ", " ", " ", " ", " ", " ", " ", " ", " ", "", " ", "", "", "", ""], [" ", " ", " ", " ", " ", " ", " ", " ", " ", " ", " ", " ", " ", " ", " ", " ", " ", " ", " ", " ", " ", " ", " ", " ", "", " ", "", "", "", ""], [" ", " ", " ", " ", " ", " ", " ", " ", " ", " ", " ", " ", " ", " ", " ", " ", " ", " ", " ", " ", " ", " ", " ", " ", "", " ", "", "", "", ""], [" ", " ", " ", " ", " ", " ", " ", " ", " ", " ", " ", " ", " ", " ", " ", " ", " ", " ", " ", " ", " ", " ", " ", " ", "", " ", "", "", "", ""], [" ", " ", " ", " ", " ", " ", " ", " ", " ", " ", " ", " ", " ", " ", " ", " ", " ", " ", " ", " ", " ", " ", " ", " ", "", " ", "", "", "", ""], [" ", " ", " ", " ", " ", " ", " ", " ", " ", " ", " ", " ", " ", " ", " ", " ", " ", " ", " ", " ", " ", " ", " ", " ", "", " ", "", "", "", ""], [" ", " ", " ", " ", " ", " ", " ", " ", " ", " ", " ", " ", " ", " ", " ", " ", " ", " ", " ", " ", " ", " ", " ", " ", "", " ", "", "", "", ""], [" ", " ", " ", " ", " ", " ", " ", " ", " ", " ", " ", " ", " ", " ", " ", " ", " ", " ", " ", " ", " ", " ", " ", " ", "", " ", "", "", "", ""], [" ", " ", " ", " ", " ", " ", " ", " ", " ", " ", " ", " ", " ", " ", " ", " ", " ", " ", " ", " ", " ", " ", " ", " ", "", " ", "", "", "", ""], ["None", "None", "None", "None", "None", "None", "None", "None", "None", "None", "None", "None", "None", "None", "None", "None", "None", "None", "None", "None", "None", "None", "None", "None", "None", "None", "", "", "", ""]]
  out "unitType":string
  out "buttonType":string
  out "pulseType":string
  out "audioType":string
  out "ConsoleVoltage":string
  out "InclineMax":string
  out "InclineMin":string
  out "TransMax":string
  out "MaxSpeed":string
  out "tempNumeric":dbl
  out "tempBoolean":bool
  out "tempString":string
  out "displayType":string
  out "mcuType":string
  out "Firmware":string
  out "Controller/PowerBoard":string
  out "deviceType":string
  out "PartNumber":string
  out "Part Name":string
  out "TV":string
  out "DEMO":string
  out "WAHOO":string
  out "CSAFE":string
  out "TABLET":string
  out "PULSE":string
  out "RESISTANCE":string
  out "BLE":string
  out "BUZZER":string
  out "AUDIO":string
  out "FAN":string
  out "DISTANCE":string
  out "GRADE":string
  out "SPEED":string
  out "DMK":string
  out "USB":string
  # "byte[0]"
  # "Form Data"
  # "byte[1]"
  # "address: 0xA9 - 0xAA MPH; 0xAB - 0xAD KPH; 0xAE - 0xB6 INC; 0xB7 - 0xBA RES; 0xBB - 0xBE GEA"
  # "bytes |----------------------------------------|----------------------------------------|-----------------------------------------|----------------------------------------|----------------------------------------|----------------------------------------|-----------------------------------------|----------------------------------------|"
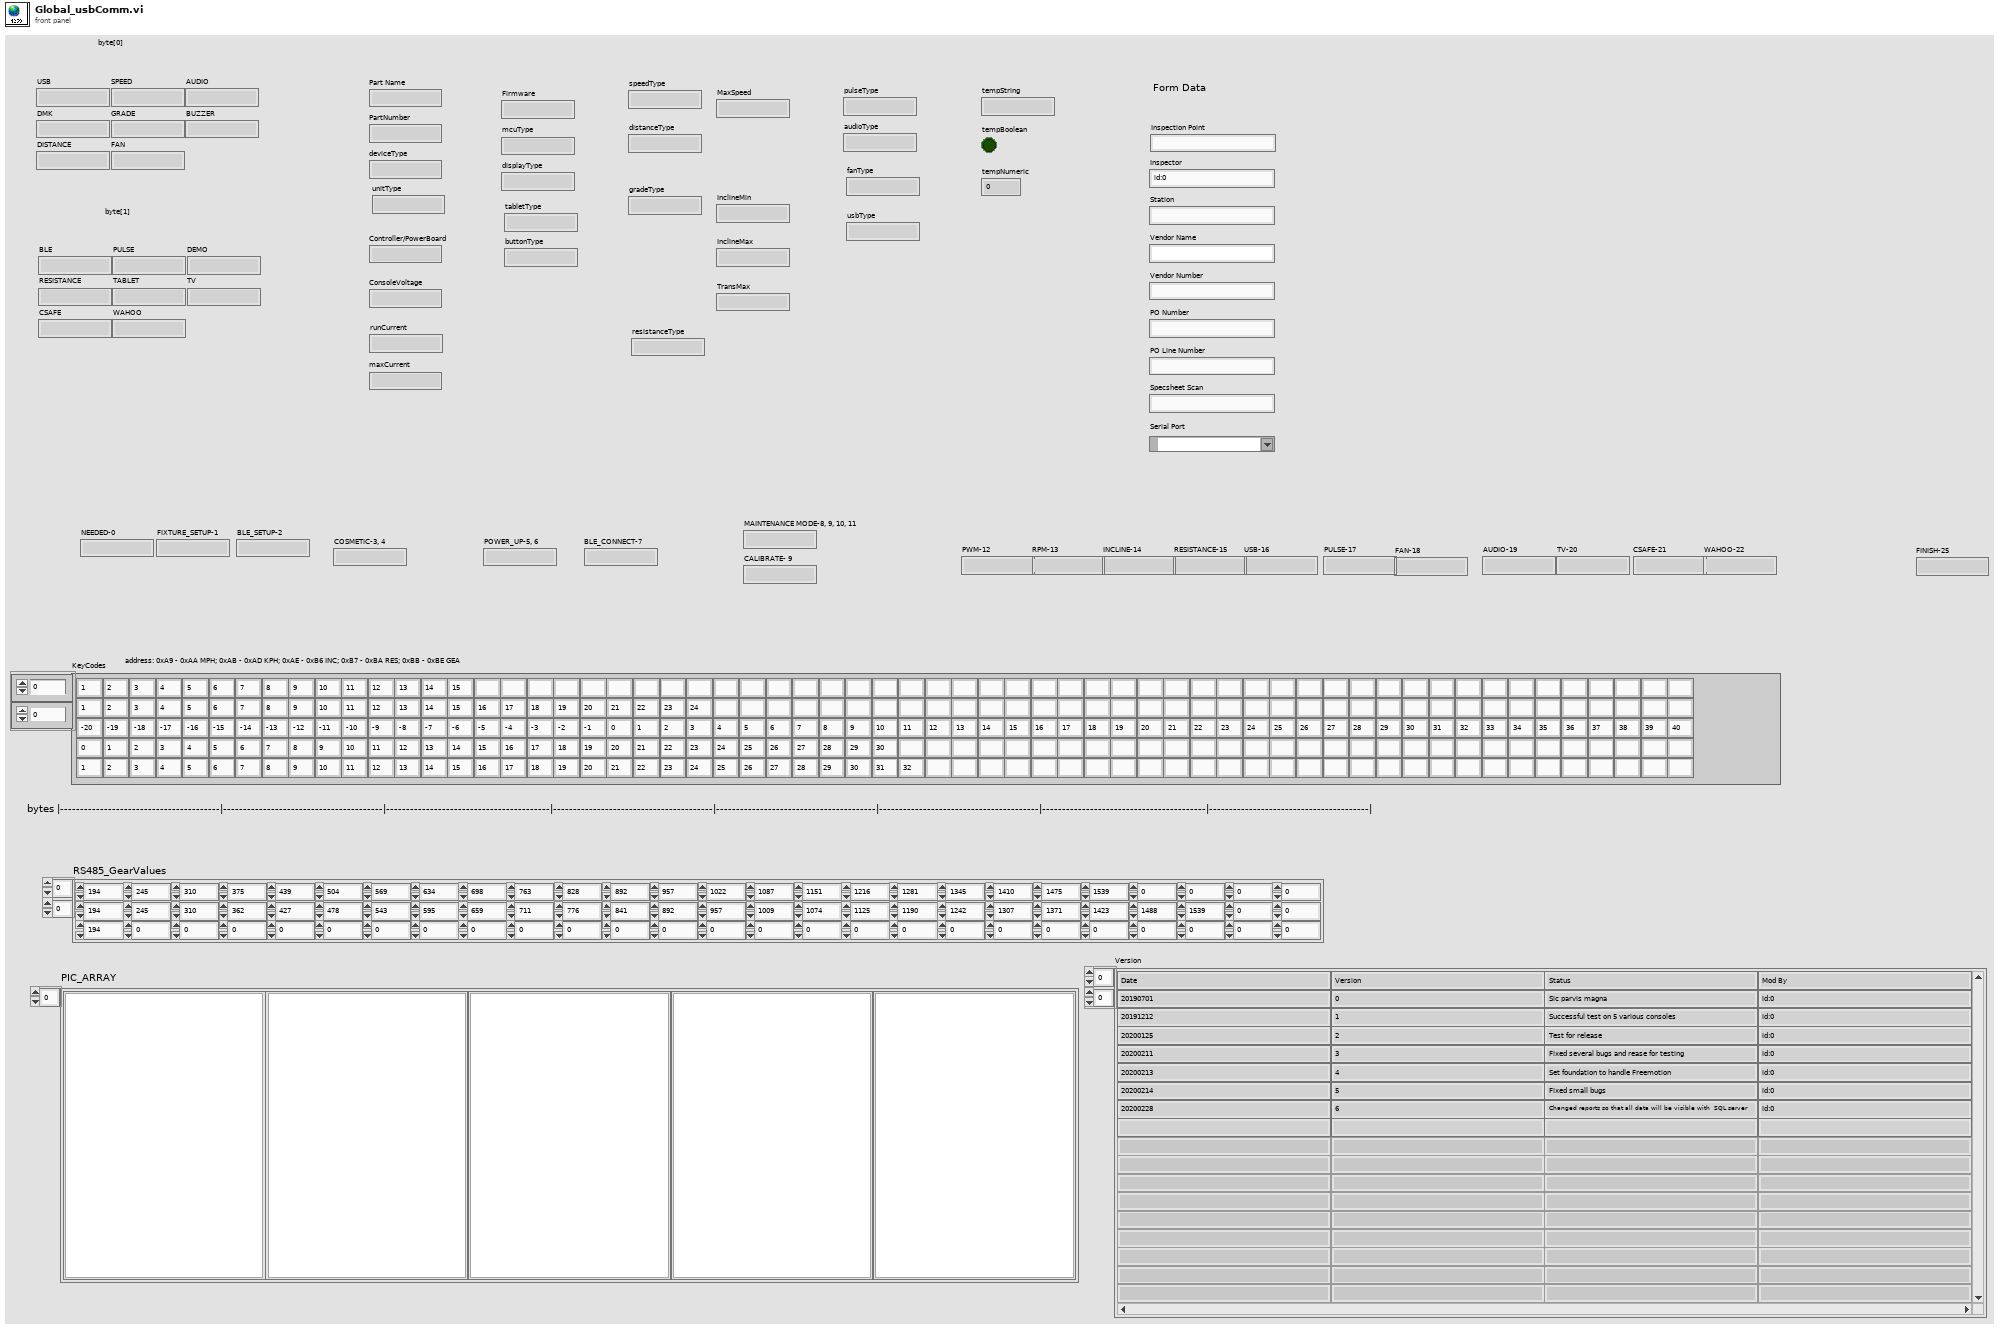
[diagram p1: front panel]
diagram:
